vi "ComplexPath.vi"() -> ()   [LabVIEW 2016, in "test_ValueSignal.lvlib"]
uses:
  test_ValueSignal.lvlib
  Helper/HelperVI1.vi
  main/apis/Setup/GetVI/GetVIByPath.vi
  main/apis/Stimulus/ValueSignal/ValueSignalByPathString.vi
  main/apis/Assert/AssertControlValue/Equal.vi
  main/apis/Setup/GetVI/GetVI.lvlib
  <vilib>/addons/_JKI Toolkits/Caraya/classes/Test/Test.lvclass
  main/apis/Assert/AssertControlValue/AssertControlValue.lvlib
panel:
  out "error out":errorcluster
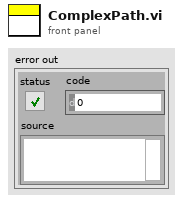
[diagram p1: front panel]
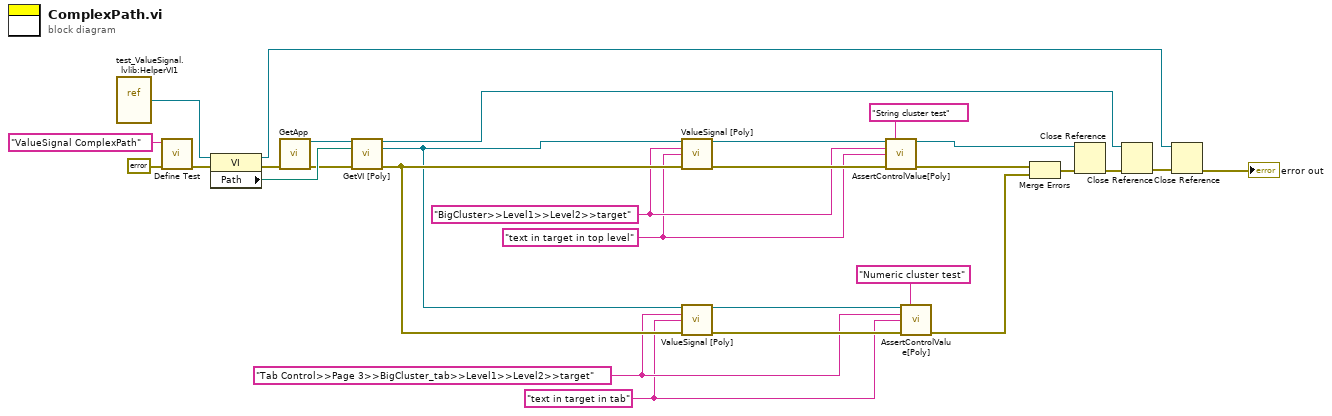
[diagram p0: block diagram]
diagram:
  w2 = "Tab Control>>Page 3>>BigCluster_tab>>Level1>>Level2>>target" ("Control Name")
  w3 = "text in target in top level" ("Control Name")
  w4 = "BigCluster>>Level1>>Level2>>target" ("Control Name")
  w1 = "text in target in tab"
  n1 = vi-ref "test_ValueSignal.lvlib:HelperVI1.vi"() -> (w5:refnum<vi>)
  n2 = call <vilib>:"Define Test.vi"("error in (no error)"=errorcluster {"status"=FALSE, "code"=0, "source"=""}, "Label (VI Title)"="ValueSignal ComplexPath") -> ("error out"=w21:errorcluster)  [unwired: 9 in]
  n3 = property on="Property Node" class="VI"(reference=w5, error in=w21) -> (reference out=w16:refnum<vi>, error out=w25:errorcluster, "Path"=w24:path)
  n4 = call "GetApp.vi"("error in (no error)"=w25) -> ("Application Ref"=w26:refnum<vi>, "error out"=w23:errorcluster)  [unwired: 13 in]
  n5 = call-poly "GetVI [Poly].vi"("Application Ref in"=w26, "VI Path"=w24, "error in (no error)"=w23) -> ("Application Ref out"=w17:refnum<vi>, "VI Reference"=w18:refnum<vi>, "error out"=w19:errorcluster)  [unwired: 10 in]
  n6 = call-poly "ValueSignal [Poly].vi"("VI Reference In"=w18, "Control Name"=w4, "Value (Signaling)"=w3, "error in"=w19) -> ("VI Reference Out"=w13:refnum<vi>, "error out"=w15:errorcluster)  [unwired: 10 in]
  n7 = call-poly "ValueSignal [Poly].vi"("VI Reference In"=w18, "Control Name"=w2, "Value (Signaling)"=w1, "error in"=w19) -> ("VI Reference Out"=w8:refnum<vi>, "error out"=w10:errorcluster)  [unwired: 10 in]
  n8 = call-poly "AssertControlValue[Poly].vi"("VI Reference In"=w13, "Label"="String cluster test" ("Label (VI Title)"), "Control Name"=w4, "Control Value"=w3, "Error In"=w15) -> ("VI Reference Out"=w12:refnum<vi>, "Error Out"=w14:errorcluster)  [unwired: 9 in]
  n9 = call-poly "AssertControlValue[Poly].vi"("VI Reference In"=w8, "Label"="Numeric cluster test" ("Label (VI Title)"), "Control Name"=w2, "Control Value"=w1, "Error In"=w10) -> ("Error Out"=w9:errorcluster)  [unwired: 9 in, 1 out]
  n10 = Merge Errors(w14, w9) -> (w27:errorcluster)
  n11 = Close Reference(reference=w12, error in (no error)=w27) -> (error out=w29:errorcluster)
  n12 = Close Reference(reference=w17, error in (no error)=w29) -> (error out=w28:errorcluster)
  n13 = Close Reference(reference=w16, error in (no error)=w28) -> (error out=→"error out":errorcluster)
